vi "Close Notebook Window Action.vi"(8 "Notebook Saved?":bool, 9 "Main VI Name":string, 11 "Notebook Queue":refnum<queue>) -> (0 "Quit?":bool)   [LabVIEW 2019, in "Notebook.lvlib"]
uses:
  Notebook.lvlib
  Notebook Action Q Element.ctl
  Notebook Action List.ctl
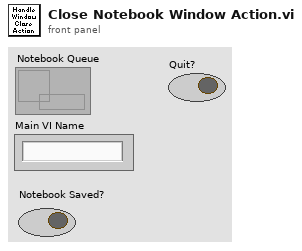
[diagram p1: front panel]
types:
  T1 = cluster{"Left Button Key Shortcut":cluster{"Control":bool, "Shift":bool, "Key":string}, "Center Button Key Shortcut":cluster{"Control":bool, "Shift":bool, "Key":string}, "Right Button Key Shortcut":cluster{"Control":bool, "Shift":bool, "Key":string}}
  T2 = enum16{"Left Button", "Center Button", "Right Button", "Window Close"}
  T3 = typedef "Notebook.lvlib/Notebook Action Q Element.ctl" = cluster{"Action":T4, "Variant":variant}
  T4 = typedef "Notebook.lvlib/Notebook Action List.ctl" = enum16{"Idle", "Init", "Check Content Change", "User added content", "Program added text", "Program added Picture ", "Save Notebook", "Quit", "Open", "Close", "Update Window Title"}
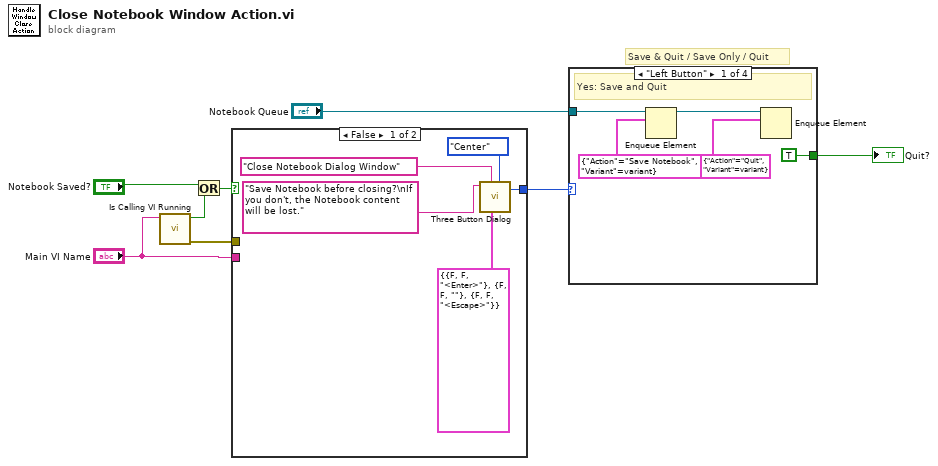
[diagram p0: block diagram]
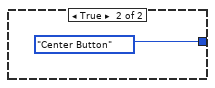
[diagram p2: hidden frame]
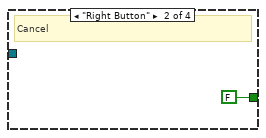
[diagram p3: hidden frame]
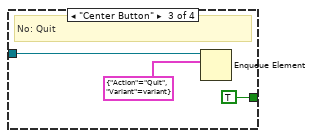
[diagram p4: hidden frame]
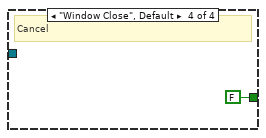
[diagram p5: hidden frame]
diagram:
  # "Save & Quit / Save Only / Quit"
  n1 = call "Is Calling VI Running.vi"("Calling VI Name"="Main VI Name") -> ("Error Out"=w1:errorcluster, "Running?"=w2:bool)  [unwired: 9 in]
  n2 = Or(x="Notebook Saved?", y=w2) -> (x .or. y?=w3:bool)
  n3 = case shown="False" w3 {
    tunnel: [w12 T2."Center Button" ("t")] -> w6
    tunnel: "Main VI Name" -> [_ _]
    tunnel: w1 -> [_ _]
    frame False {
      n4 = call <vilib>:"Three Button Dialog.vi"("Justify Message (Left)"=enum16{"Left", "Center", "Right"}."Center", "Keyboard Shortcuts (Left is <Enter>)"=T1 {"Left Button Key Shortcut"={"Control"=FALSE, "Shift"=FALSE, "Key"="<Enter>"}, "Center Button Key Shortcut"={"Control"=FALSE, "Shift"=FALSE, "Key"=""}, "Right Button Key Shortcut"={"Control"=FALSE, "Shift"=FALSE, "Key"="<Escape>"}}, "Window Title (\"\")"="Close Notebook Dialog Window" ("Window Title (\"\")"), "message"="Save Notebook before closing?\nIf you don't, the Notebook content will be lost.") -> ("Which Button?"=w12:T2)  [unwired: 7 in]
    }
    frame True {
    }
  }
  n5 = case shown="\"Left Button\"" w6 {
    tunnel: "Notebook Queue" -> [w19 _ w23 _]
    tunnel: [TRUE ("Discard?") FALSE ("Discard?") TRUE ("Discard?") FALSE ("Discard?")] -> w7
    frame "Left Button" {
      # "Yes: Save and Quit"
      n6 = Enqueue Element(queue=w19, element=T3 {"Action"=enum."Save Notebook", "Variant"=variant}) -> (queue out=w17:refnum<queue>)  [unwired: 2 in, 2 out]
      n7 = Enqueue Element(queue=w17, element=T3 {"Action"=enum."Quit", "Variant"=variant}) -> ()  [unwired: 2 in, 3 out]
    }
    frame "Right Button" {
      # "Cancel"
    }
    frame "Center Button" {
      # "No: Quit"
      n8 = Enqueue Element(queue=w23, element=T3 {"Action"=enum."Quit", "Variant"=variant}) -> ()  [unwired: 2 in, 3 out]
    }
    frame "Window Close", Default {
      # "Cancel"
    }
  }
  "Quit?" <- w7
